vi "FG_FPGA_Interface.vi"(7 "Action":T1, 8 "error in":errorcluster) -> (0 "error out":errorcluster)   [LabVIEW 2013]
uses:
  Typedef_FPGA_Interface_Action.ctl
  <vilib>/rvi/interface/common/niFpgaWaitOnOcc.vi
  <vilib>/nisyscfg/Initialize (Control).vi
  <vilib>/nisyscfg/Find Hardware.vi
  <vilib>/FPGAPlugInAG/sbRIO-9606/niLvFpga_Open_sbRIO-9606.vi
  <vilib>/rvi/interface/common/dynamic/niFpgaDynamicAddResources.vi
  <vilib>/Utility/error.llb/Error Cluster From Error Code.vi
  <vilib>/rvi/errors/niLvFpgaAdjustHostInterfaceError.vi
  <vilib>/FPGAPlugInAG/Dynamic/niLvFpga_Close_Dynamic.vi
  <vilib>/rvi/interface/nirviOpenFPGA/nirviOpenFPGA.xnode
  FPGA Bitfiles/8-AxisKNR.lvbitx
  <vilib>/rvi/interface/nirviReadWriteControl/nirviReadWriteControl.xnode
  <vilib>/rvi/interface/nirviCloseFPGA/nirviCloseFPGA.xnode
  <vilib>/nisyscfg/nisyscfg.lvlib
  <vilib>/rvi/interface/Simulation/niFpgaSimulationCallBeginRW.vi
  NiFpgaLv.dll
panel:
  out "Numeric":i32
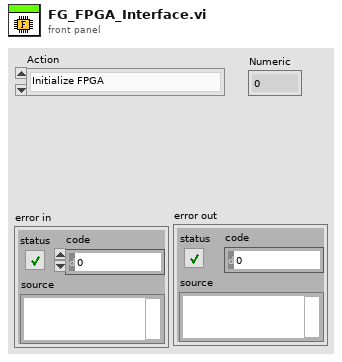
[diagram p1: front panel]
types:
  T1 = typedef "Typedef_FPGA_Interface_Action.ctl" = enum16{"Initialize FPGA", "Get FPGA Reference", "Close FPGA"}
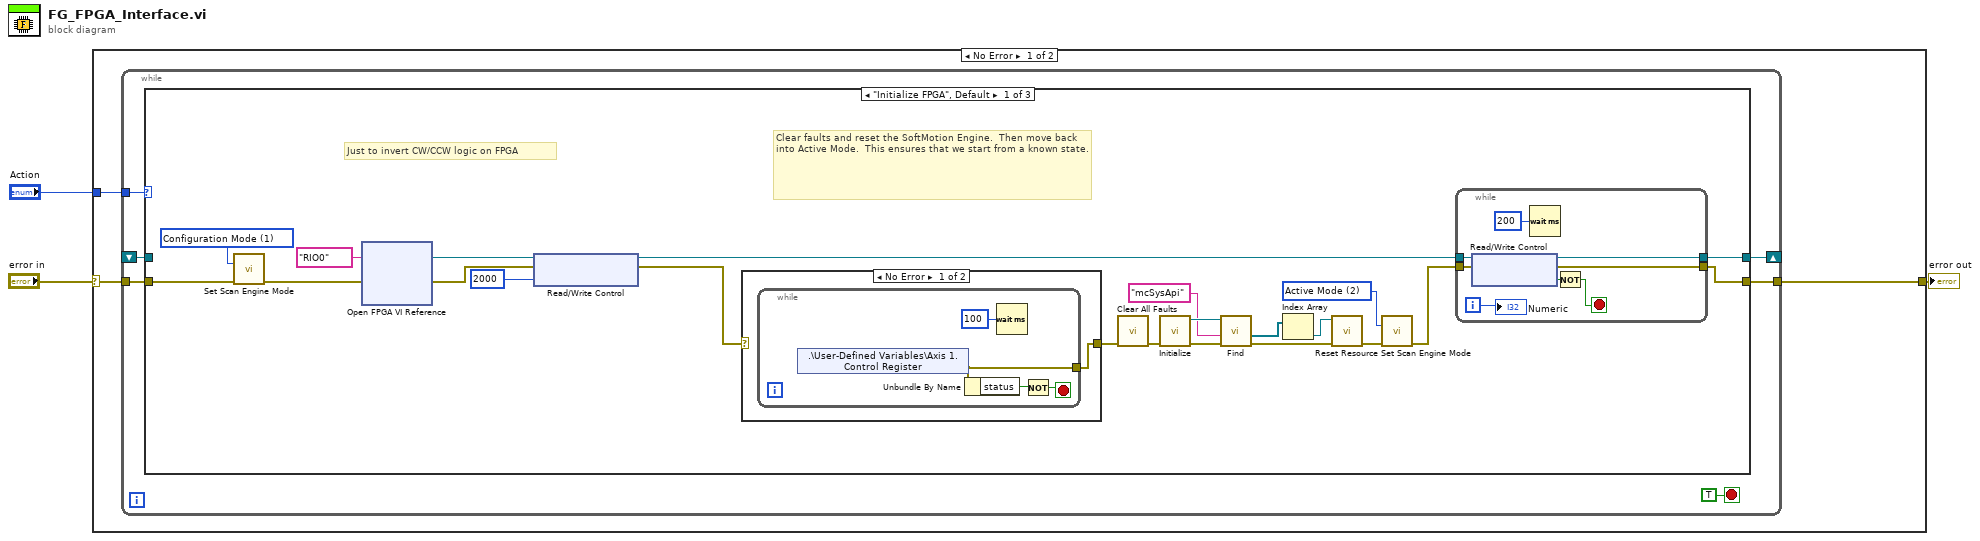
[diagram p0: block diagram]
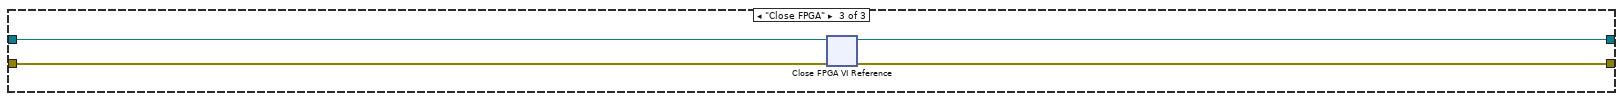
[diagram p4: hidden frame]
diagram:
  n1 = case shown="No Error" "error in" {
    selector: "error in" -> [w6 w54]
    tunnel: [w5 w54] -> w2
    tunnel: "Action" -> [w4 _]
    frame No Error {
      n2 = while {
        tunnel: w6 -> [w10]
        tunnel: w4 -> [w11]
        tunnel: [w9] -> w5
        shift-right: [w8] -> _
        shift-left: _ -> [w7]
        stop <- TRUE stop-if-true
        n3 = case shown="\"Initialize FPGA\", Default" w11 {
          tunnel: w10 -> [w33 w49 w52]
          tunnel: [w15 w49 w53] -> w9
          tunnel: w7 -> [_ w50 w51]
          tunnel: [w16 w50 w51] -> w8
          frame "Initialize FPGA", Default {
            w18 = 2 items=["Configuration Mode"=1, "Active Mode"=2] ("mode (Active Mode)")
            w27 = 1 items=["Configuration Mode"=1, "Active Mode"=2] ("mode (Active Mode)")
            # "Just to invert CW/CCW logic on FPGA"
            # "Clear faults and reset the SoftMotion Engine.  Then move back into Active Mode.  This ensures that we start from a known state."
            n4 = call <vilib>:"Set Scan Engine Mode.vi"("mode (Active Mode)"=w27, "error in (no error)"=w33) -> ("error out"=w32:errorcluster)  [unwired: 13 in]
            n5 = xnode "Open FPGA VI Reference"("error in"=w32, "resource name"=tag "RIO0") -> ("FPGA VI Reference Out"=w13:refnum<k20>, "error out"=w14:errorcluster)
            n6 = xnode "Read/Write Control"("FPGA VI Reference In"=w13, "error in"=w14, "minimum pulse"=u16 2000) -> ("FPGA VI Reference Out"=w17:refnum<k20>, "error out"=w30:errorcluster)
            n7 = case shown="No Error" w30 {
              selector: w30 -> [_ w48]
              tunnel: [w43 w48] -> w31
              frame No Error {
                n8 = while {
                  tunnel: [w44] -> w43
                  stop <- w47 stop-if-true
                  n9 = shared-variable ".\\User-Defined Variables\\Axis 1.Control Register"() -> (error out=w44:errorcluster)  [unwired: 1 in, 1 out]
                  n10 = Unbundle By Name(w44) -> ("status"=w46:bool)
                  n11 = Wait (ms)(milliseconds to wait=u32 100) -> ()  [unwired: 1 out]
                  n12 = Not(x=w46) -> (.not. x?=w47:bool)
                }
              }
              frame Error {
              }
            }
            n13 = call <vilib>:"Clear All Faults.vi"("error in (no error)"=w31) -> ("error out"=w25:errorcluster)  [unwired: 10 in]
            n14 = call-poly <vilib>:"Initialize.vi"("error in (no error)"=w25) -> ("error out"=w19:errorcluster, "session out"=w21:refnum<k21>)  [unwired: 8 in, 1 out]
            n15 = call-poly <vilib>:"Find.vi"("error in (no error)"=w19, "experts"="mcSysApi", "session in"=w21) -> ("error out"=w24:errorcluster, "resources out"=w22:refnum<k20>[])  [unwired: 5 in, 2 out]
            n16 = Index Array(array=w22) -> (element=w23:refnum<k20>)  [unwired: 1 in]
            n17 = call <vilib>:"Reset Resource.vi"("error in (no error)"=w24, "resource in"=w23) -> ("error out"=w26:errorcluster)  [unwired: 8 in, 1 out]
            n18 = call <vilib>:"Set Scan Engine Mode.vi"("mode (Active Mode)"=w18, "error in (no error)"=w26) -> ("error out"=w29:errorcluster)  [unwired: 13 in]
            n19 = while {
              tunnel: w29 -> [w42]
              tunnel: [w41] -> w15
              tunnel: w17 -> [w37]
              tunnel: [w36] -> w16
              i -> [w35]
              stop <- w38 stop-if-true
              n20 = xnode "Read/Write Control"("FPGA VI Reference In"=w37, "error in"=w42) -> ("FPGA VI Reference Out"=w36:refnum<k20>, "error out"=w41:errorcluster, "Sync is Fault"=w40:bool)
              n21 = Wait (ms)(milliseconds to wait=u32 200) -> ()  [unwired: 1 out]
              n22 = Not(x=w40) -> (.not. x?=w38:bool)
              "Numeric" <- w35
            }
          }
          frame "Get FPGA Reference" {
          }
          frame "Close FPGA" {
            n23 = xnode "Close FPGA VI Reference"("FPGA VI Reference In"=w51, "error in"=w52) -> ("error out"=w53:errorcluster)
          }
        }
      }
    }
    frame Error {
    }
  }
  "error out" <- w2
